vi "HandleError.vi"(8 "error in (no error)":errorcluster, 11 "queue":refnum<queue>) -> (0 "error out":errorcluster, 3 "queue out":refnum<queue>)   [LabVIEW 2019, in "ManualMode.lvlib"]
uses:
  ManualMode.lvlib
  Cluster - ManualModeMessageCluster.ctl
  Enum - ManualModeMessage.ctl
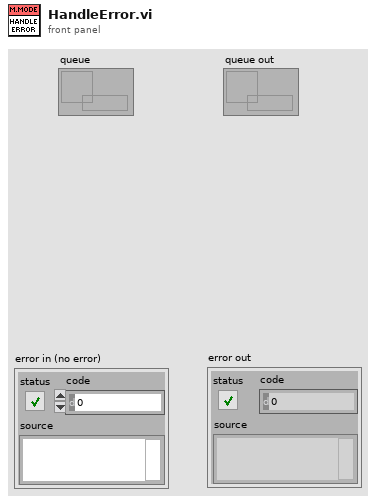
[diagram p1: front panel]
types:
  T1 = typedef "ManualMode.lvlib/Enum - ManualModeMessage.ctl" = enum16{"Initialize", "Idle", "Start", "Stop", "Pause", "Resume", "BroadcastPreCollection", "MoveCCW", "MoveCW", "StopMove", "SetZero", "GotoZero", "UpdateHW", "SendMark10Cmd", "ReadPosition", "ReadTorque", "ReadStatus", "Error", "Exit"}
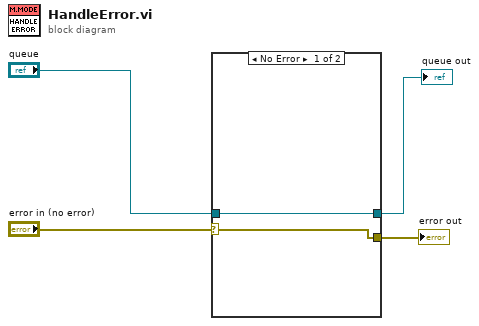
[diagram p0: block diagram]
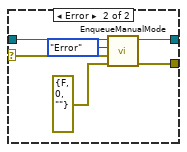
[diagram p2: hidden frame]
diagram:
  n1 = case shown="No Error" "error in (no error)" {
    selector: "error in (no error)" -> [w5 w9]
    tunnel: [w5 w12] -> w4
    tunnel: "queue" -> [w6 w11]
    tunnel: [w6 w10] -> w2
    frame No Error {
    }
    frame Error {
      n2 = call "EnqueueManualMode.vi"("error in (no error)"=errorcluster {"status"=FALSE, "code"=0, "source"=""}, "Data"=w9, "Message"=Enum_-_ManualModeMessage."Error", "queue"=w11) -> ("error out"=w12:errorcluster, "queue out"=w10:refnum<queue>)  [unwired: 6 in]
    }
  }
  "error out" <- w4
  "queue out" <- w2
